vi "simple_qa_agent_sm_template.vi"() -> ()   [LabVIEW 2020]
uses:
  user_interfaces/simple_html_chat_ui/simple_html_chat_ui.lvclass
  models/abstract_llm_base/abstract_llm_base.lvclass
  vectorstore/abstract_vector_base/abstract_vector_base.lvclass
  agent_simple_qa/agent_simple_qa.lvclass
  models/message_text/message_text.lvclass
  <vilib>/addons/_JKI Toolkits/State Machine/_JKI_lib_State_Machine.llb/Select State(s)_err__jki_lib_state_machine.vi
  vectorstore/vector_qdrant/vector_qdrant.lvclass
  D:/petwork/labview-llm-libraries/src/vectorstore/abstract_vector_base/abstract_vector_base.lvclass
  models/llm_openai_chatmodels/llm_openai_chatmodels.lvclass
  D:/petwork/labview-llm-libraries/src/models/abstract_llm_base/abstract_llm_base.lvclass
  models/llm_openai_embedding/llm_openai_embedding.lvclass
  agent_simple_qa_dynamicdata/agent_simple_qa_dynamic.lvclass
  D:/petwork/labview-llm-libraries/src/agent/agent_simple_qa/agent_simple_qa.lvclass
  <vilib>/addons/_JKI Toolkits/State Machine/_JKI_lib_State_Machine.llb/Periodic Trigger__ogtk__JKI-SM__jki_lib_state_machine.vi
  models/message_text/create_text_message.vi
  models/llm_openai_chatmodels/Instantiate_llm_openai.vi
  models/llm_openai_embedding/Instantiate_llm_openai_embed.vi
  agent_simple_qa/poly/ask_your_model.vi
panel:
  in  "new_message":string
  in  "send":bool
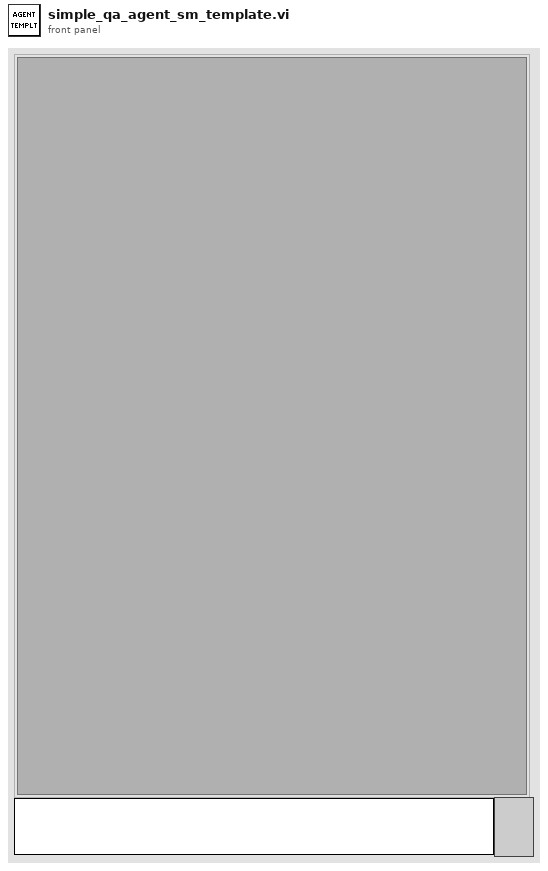
[diagram p1: front panel]
types:
  T1 = enum32{"Invalid", "Standard", "Closed", "Hidden", "Minimized", "Maximized"}
  T2 = enum32{"invalid app kind", "Development System", "Run Time System", "Student Edition", "Embedded LabVIEW", "Evaluation", "Custom"}
  T3 = cluster{"Core":cluster{"Current VI Reference":refnum<vi>, "Close Panel on Exit?":bool}, "Agent":cluster{"UI_Chat":refnum<class "simple_html_chat_ui.lvclass">, "Model_Generative":refnum<class "abstract_llm_base.lvclass">, "Model_Embedding":refnum<class "abstract_llm_base.lvclass">, "Vector Store":refnum<class "abstract_vector_base.lvclass">, "Agent_QA":refnum<class "agent_simple_qa.lvclass">, "last_message":refnum<class "message_text.lvclass">}}
  T4 = cluster{"UI_Chat":refnum<class "simple_html_chat_ui.lvclass">, "Model_Generative":refnum<class "abstract_llm_base.lvclass">, "Model_Embedding":refnum<class "abstract_llm_base.lvclass">, "Vector Store":refnum<class "abstract_vector_base.lvclass">, "Agent_QA":refnum<class "agent_simple_qa.lvclass">, "last_message":refnum<class "message_text.lvclass">}
  T5 = cluster{"Current VI Reference":refnum<vi>, "Close Panel on Exit?":bool}
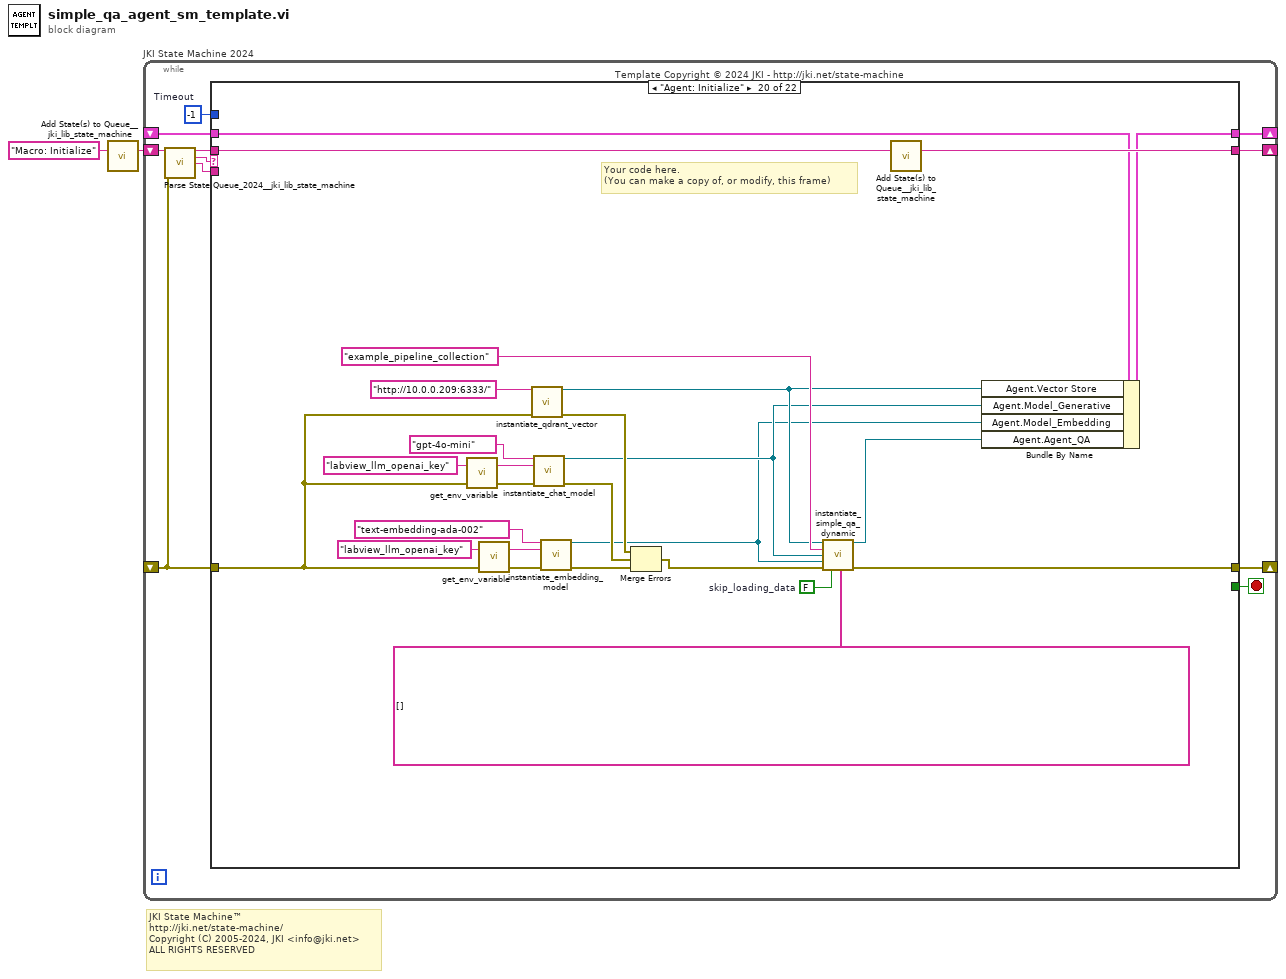
[diagram p0: block diagram]
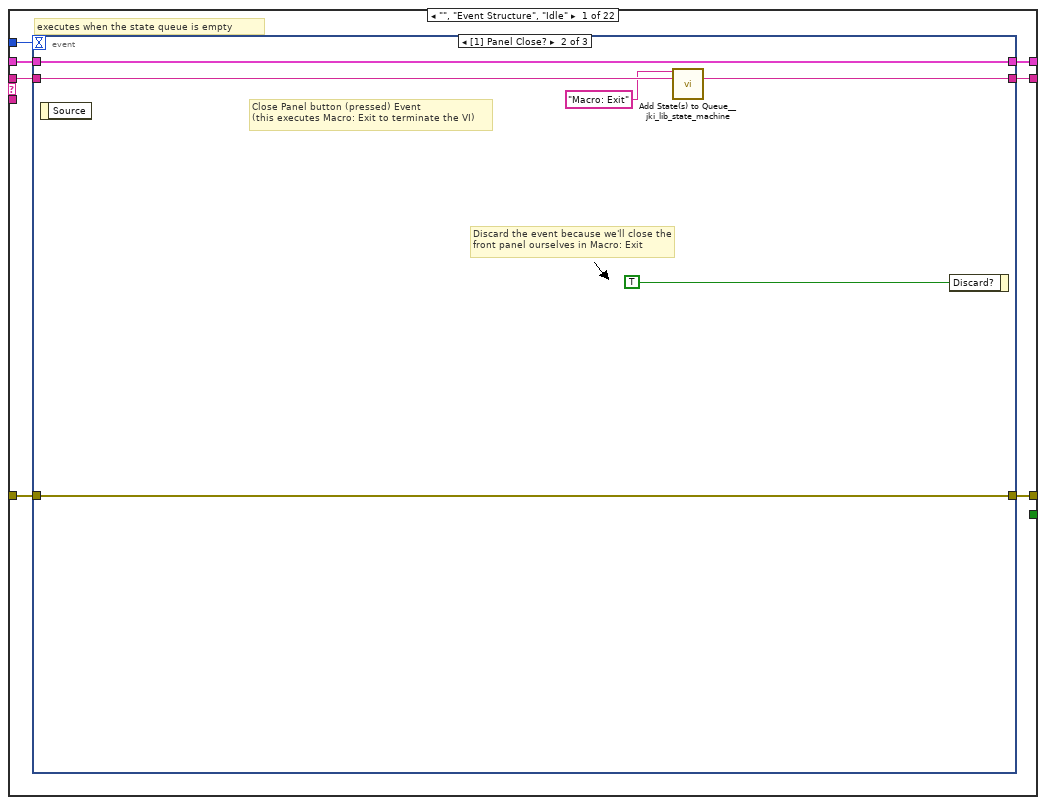
[diagram p2: hidden frame]
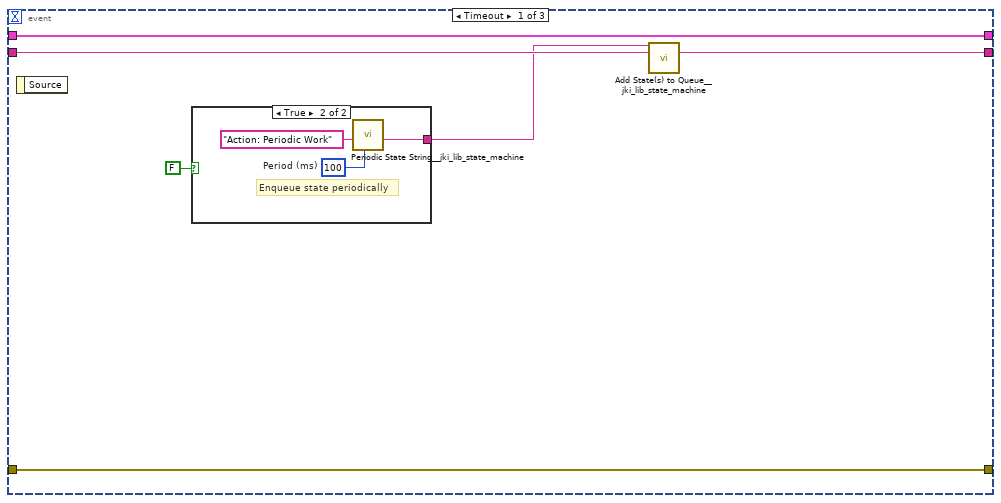
[diagram p3: hidden frame]
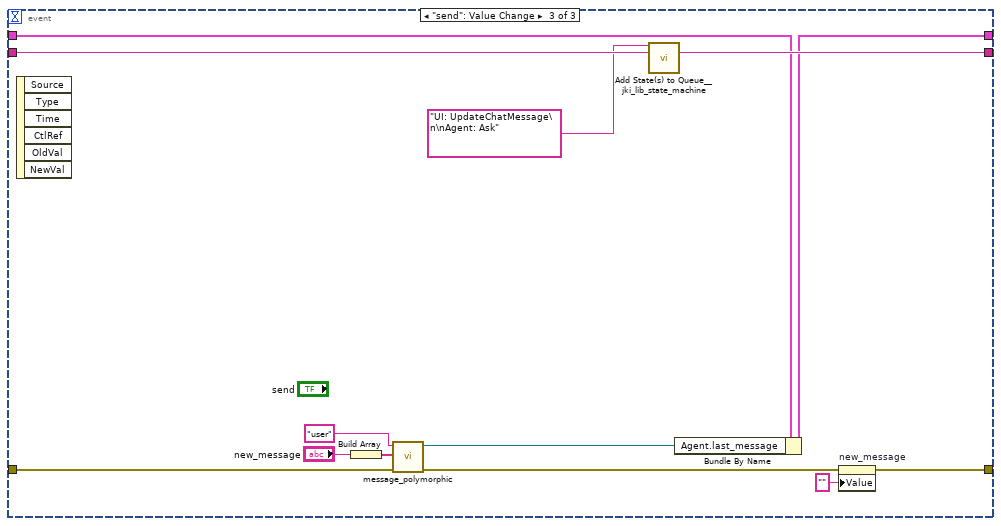
[diagram p5: hidden frame]
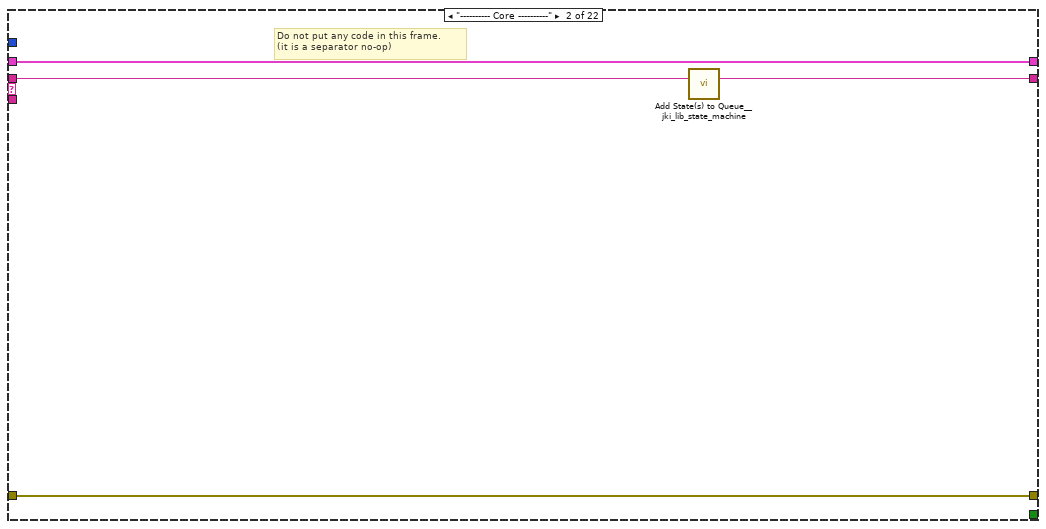
[diagram p6: hidden frame]
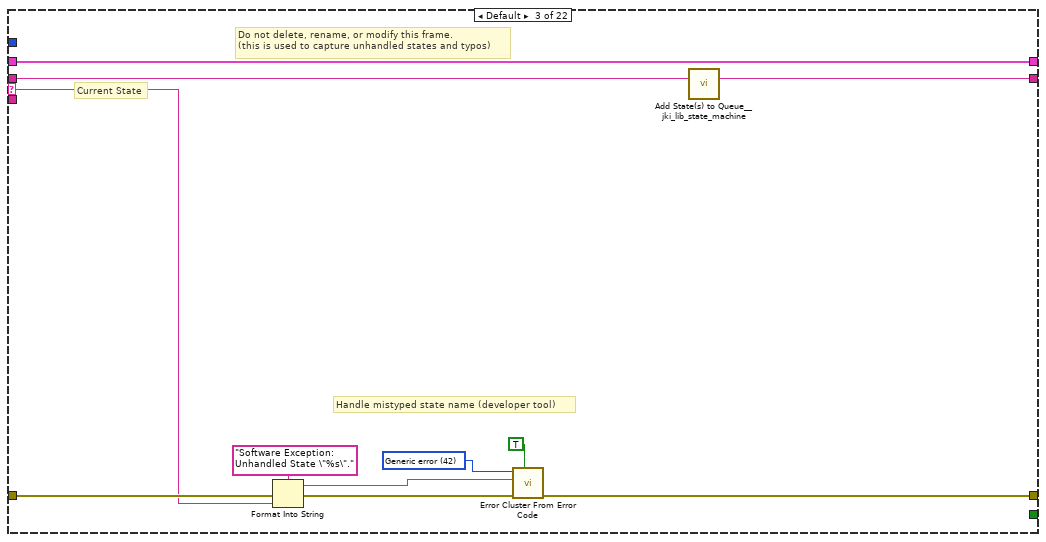
[diagram p7: hidden frame]
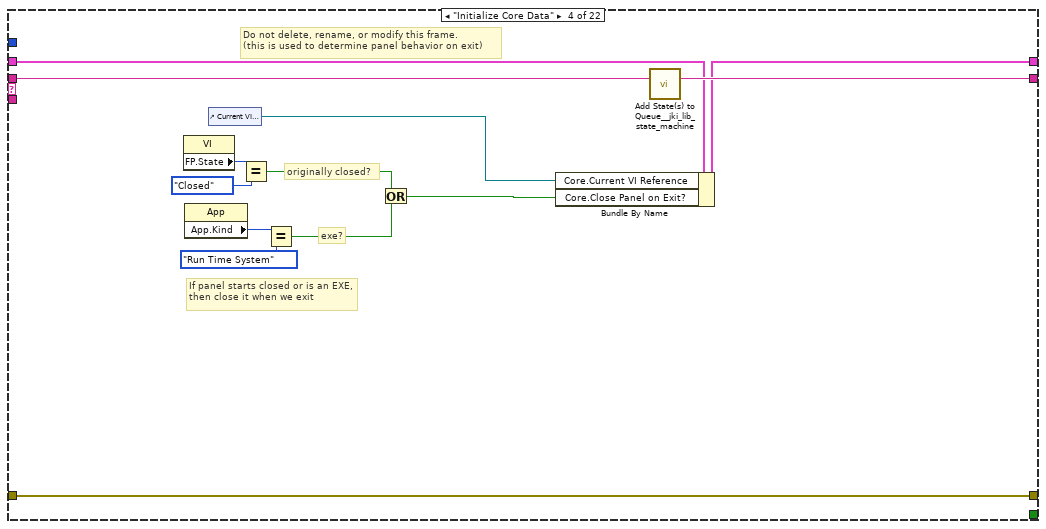
[diagram p8: hidden frame]
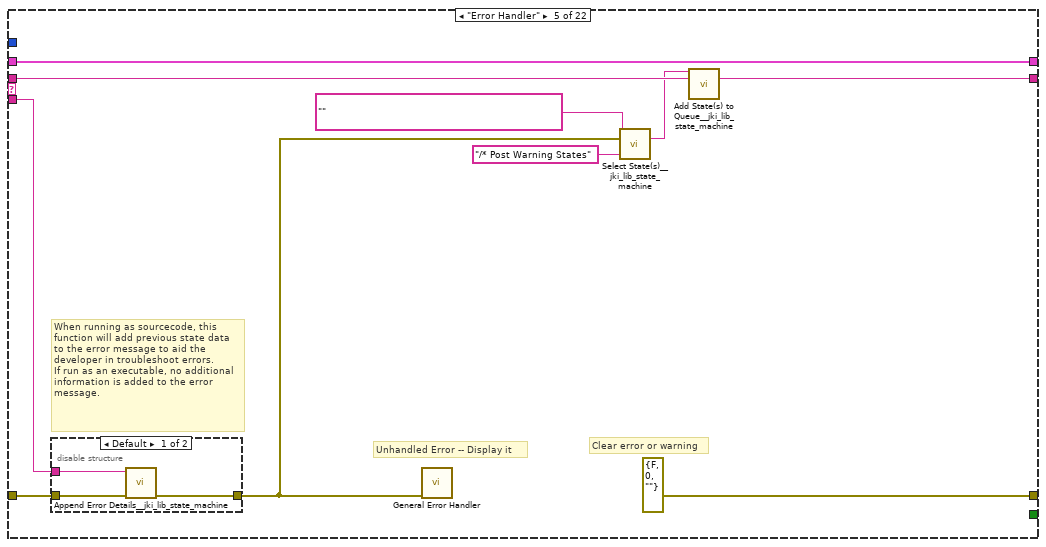
[diagram p9: hidden frame]
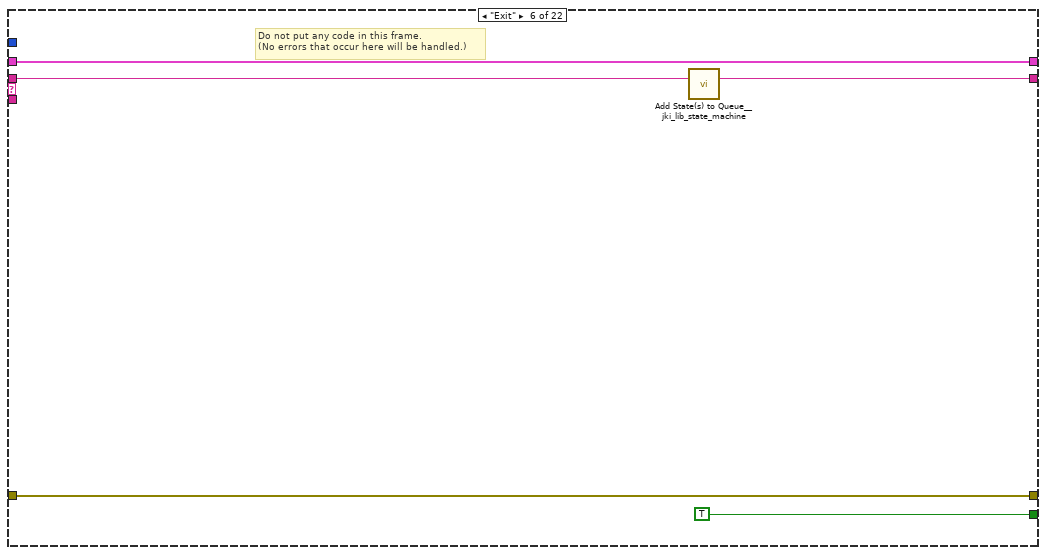
[diagram p11: hidden frame]
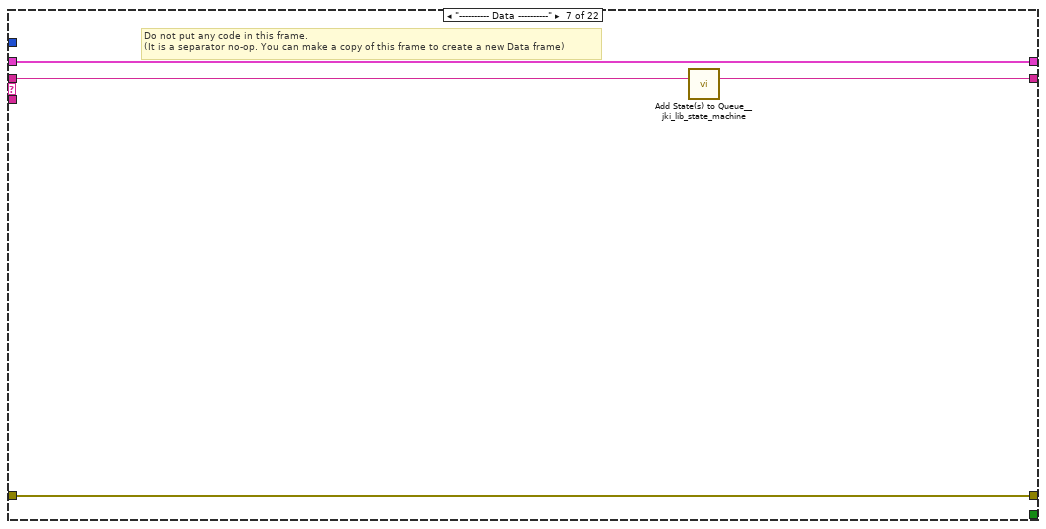
[diagram p12: hidden frame]
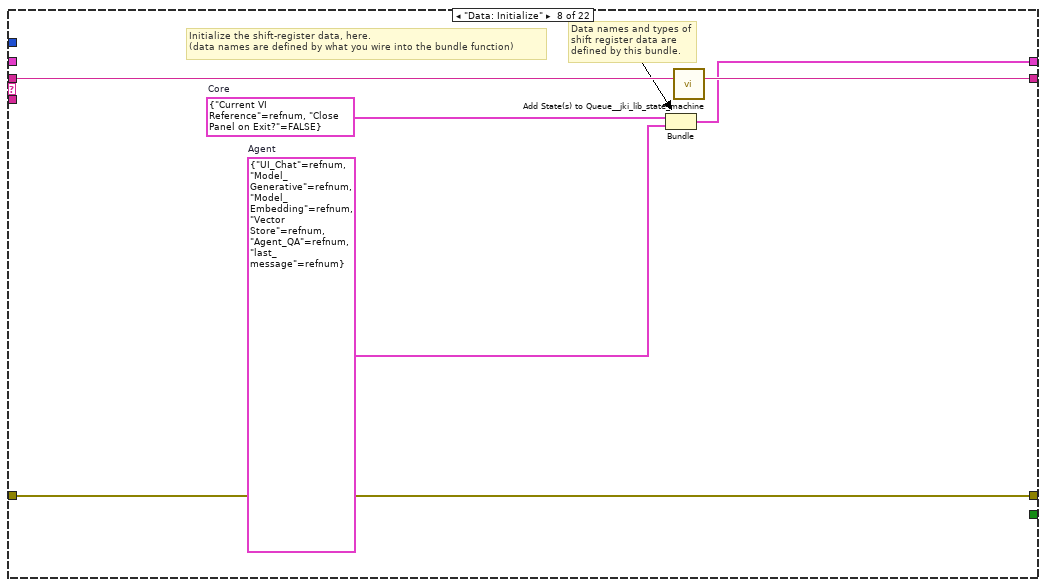
[diagram p13: hidden frame]
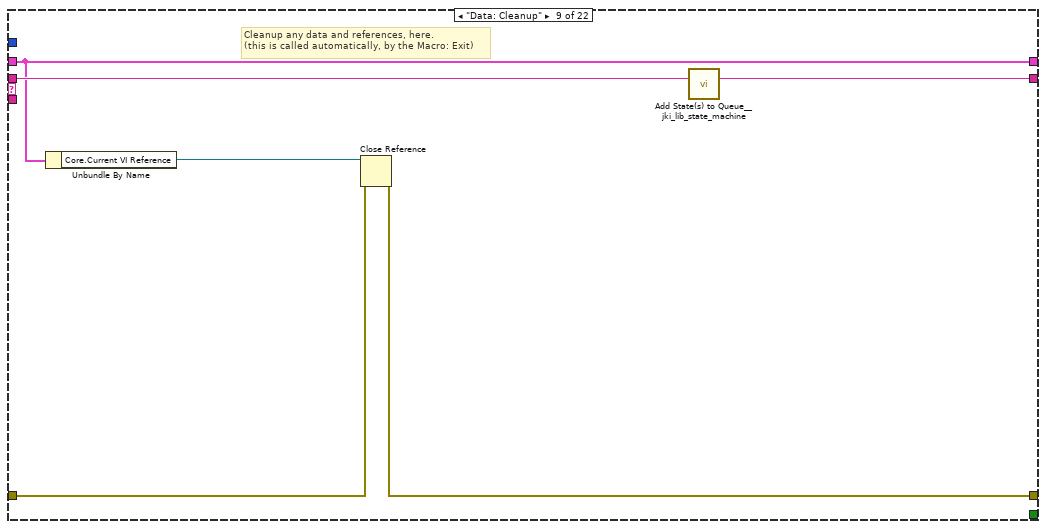
[diagram p14: hidden frame]
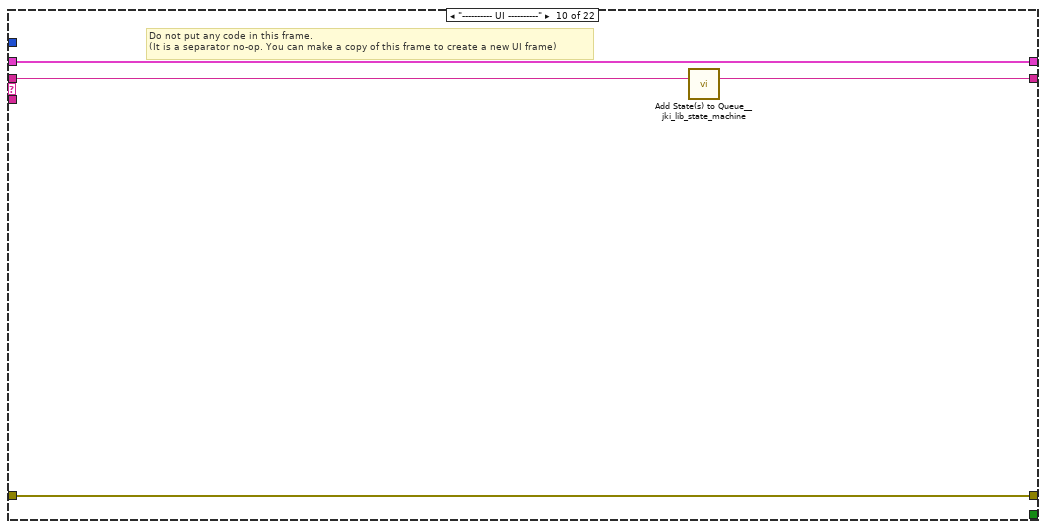
[diagram p15: hidden frame]
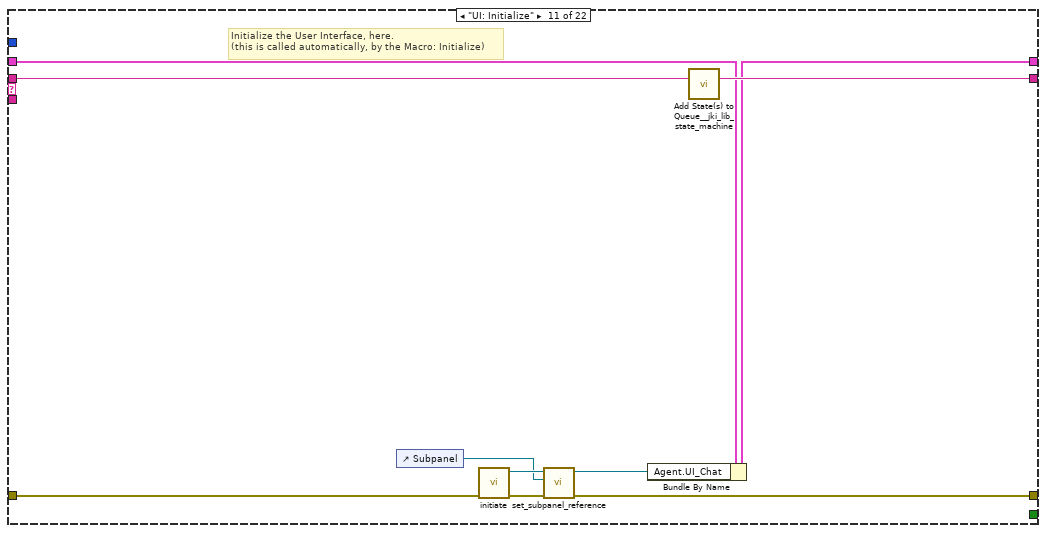
[diagram p16: hidden frame]
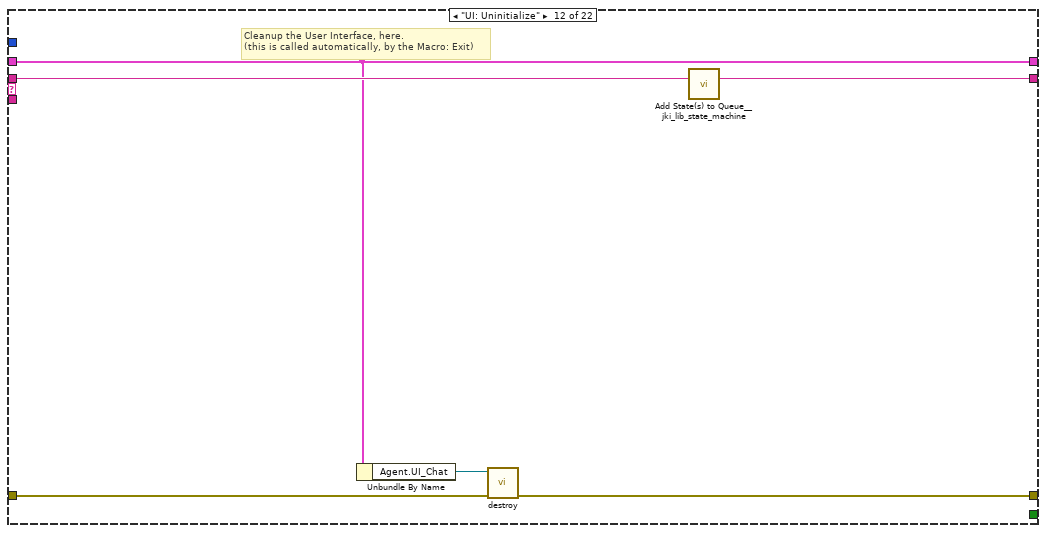
[diagram p17: hidden frame]
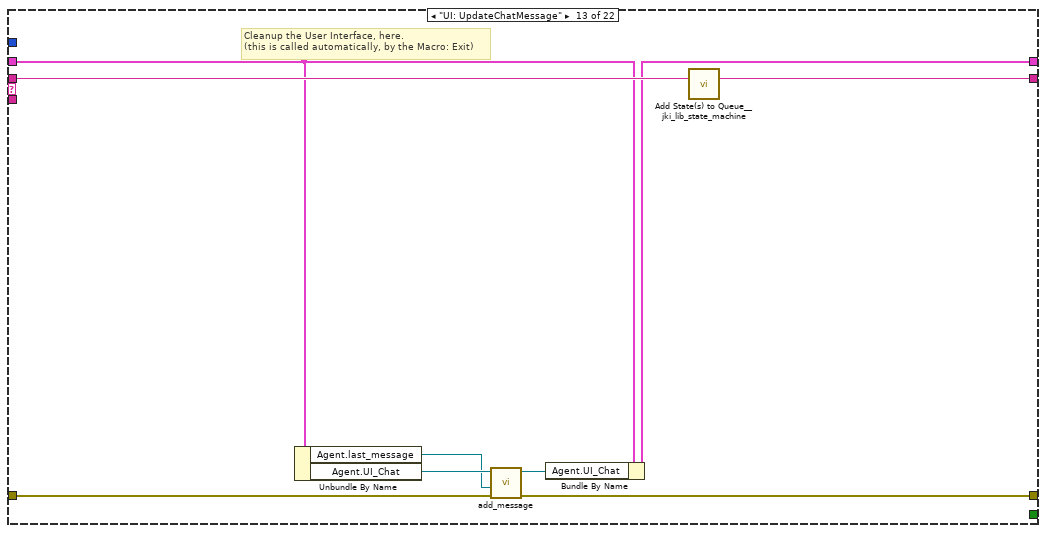
[diagram p18: hidden frame]
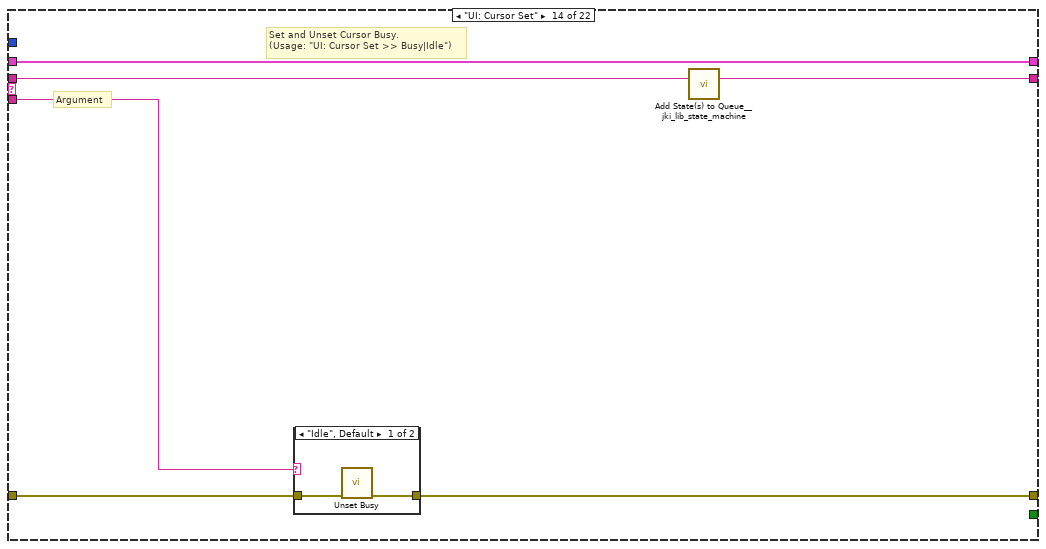
[diagram p19: hidden frame]
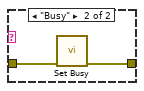
[diagram p20: hidden frame]
diagram:
  # "JKI State Machine™\nhttp://jki.net/state-machine/\nCopyright (C) 2005-2024, JKI <info@jki.net>\nALL RIGHTS RESERVED"
  n1 = call <vilib>:"Add State(s) to Queue__jki_lib_state_machine.vi"("State(s) in (\"\")"="Macro: Initialize") -> ("States Out"=w2:string)  [unwired: 14 in]
  n2 = while "JKI State Machine 2024" {
    shift-right: [w6] -> _
    shift-left: _ -> [w5]
    shift-right: [w9] -> _
    shift-left: _ -> [w3]
    shift-right: [w8] -> _
    shift-left: w2 -> [w10]
    stop <- w7 stop-if-true
    w4 = -1  # Timeout
    # "Template Copyright © 2024 JKI - http://jki.net/state-machine"
    n3 = call <vilib>:"Parse State Queue_2024__jki_lib_state_machine.vi"("State Queue"=w10, "Error In (no error)"=w3) -> ("Remaining States"=w12:string, "Current State"=w13:string, "Arguments"=w11:string)  [unwired: 11 in]
    n4 = case shown="\"Agent: Initialize\"" w13 {
      selector: w13 -> [_ _ w53 _ _ _ _ _ _ _ _ _ _ _ _ _ _ _ _ _ _ _]
      tunnel: w12 -> [w20 w52 w57 w76 w86 w95 w99 w105 w111 w115 w125 w131 w140 w146 w157 w226 w231 w240 w244 w268 w280 w291]
      tunnel: w11 -> [_ _ _ _ w82 _ _ _ _ _ _ _ _ w141 w151 _ _ _ _ _ _ _]
      tunnel: w5 -> [w18 w49 w55 w69 w77 w93 w96 _ w106 w112 w118 w129 w135 w144 w153 w223 w228 w238 w241 w250 w278 w286]
      tunnel: [w17 w50 w59 w73 errorcluster {"status"=FALSE, "code"=0, "source"=""} ("error out") w92 w97 w102 w107 w113 w119 w127 w137 w142 w154 w224 w229 w235 w242 w256 w272 w287] -> w9
      tunnel: w3 -> [w14 w50 w58 w73 w83 w92 w97 w102 w108 w113 w120 w128 w138 w143 w155 w224 w229 w235 w242 w254 w276 w288]
      tunnel: [w19 w51 w56 w75 w85 w94 w98 w104 w110 w114 w124 w130 w139 w145 w156 w225 w230 w239 w243 w267 w279 w290] -> w8
      tunnel: [_ _ _ _ _ TRUE _ _ _ _ _ _ _ _ _ _ _ _ _ _ _ _] -> w7
      tunnel: [w16 w49 w55 w74 w77 w93 w96 w103 w106 w112 w117 w129 w134 w144 w153 w223 w228 w238 w241 w249 w278 w284] -> w6
      tunnel: w4 -> [w15 _ _ _ _ _ _ _ _ _ _ _ _ _ _ _ _ _ _ _ _ _]
      frame "", "Event Structure", "Idle" {
        # "executes when the state queue is empty"
        n5 = event shown="[1] Panel Close?" {
          selector: _ -> [_ _ _]
          dyn-events: _ -> [_ _ _]
          timeout: w15 -> [_ _ _]
          tunnel: w20 -> [w26 w35 w48]
          tunnel: [w25 w34 w47] -> w19
          tunnel: w18 -> [w23 w32 w41]
          tunnel: [w24 w33 w37] -> w17
          tunnel: w14 -> [w24 w33 w43]
          tunnel: [w23 w32 w39] -> w16
          event Timeout {
            n6 = event-data() -> ()  [unwired: 1 in, 1 out]
            n7 = case shown="True" FALSE {
              tunnel: [_ w29] -> w22
              frame False {
              }
              frame True {
                w27 = u32 100  # Period (ms)
                # "Enqueue state periodically"
                n8 = call <vilib>:"Periodic State String__jki_lib_state_machine.vi"("Period (ms)"=w27, "State"="Action: Periodic Work") -> ("State Out"=w29:string)  [unwired: 9 in]
              }
            }
            n9 = call <vilib>:"Add State(s) to Queue__jki_lib_state_machine.vi"("State(s) in Front (\"\")"=w22, "State(s) in (\"\")"=w26) -> ("States Out"=w25:string)  [unwired: 13 in]
          }
          event Panel Close? {
            # "Discard the event because we'll close the front panel ourselves in Macro: Exit"
            # "Close Panel button (pressed) Event\n(this executes Macro: Exit to terminate the VI)"
            n10 = event-data() -> ()  [unwired: 1 in, 1 out]
            n11 = call <vilib>:"Add State(s) to Queue__jki_lib_state_machine.vi"("State(s) in Front (\"\")"="Macro: Exit", "State(s) in (\"\")"=w35) -> ("States Out"=w34:string)  [unwired: 13 in]
            n12 = event-data("Discard?"=TRUE) -> ()  [unwired: 1 in, 1 out]
          }
          event "send": Value Change {
            n13 = event-data() -> ()  [unwired: 1 in, 6 out]
            n14 = Build Array("new_message") -> (w44:string[])
            n15 = call-poly "message_polymorphic.vi"("error in (no error)"=w43, "content"=w44, "role"="user") -> ("error out"=w38:errorcluster, "message_text out"=w40:refnum<class "message_text.lvclass">)  [unwired: 7 in]
            n16 = call <vilib>:"Add State(s) to Queue__jki_lib_state_machine.vi"("State(s) in Front (\"\")"="UI: UpdateChatMessage\n\nAgent: Ask", "State(s) in (\"\")"=w48) -> ("States Out"=w47:string)  [unwired: 13 in]
            n17 = Bundle By Name(cluster=w41, "Agent.last_message"=w40) -> (w39:T3)
            n18 = property on="new_message" class="Str"(error in=w38, "Value"="" ("new_message")) -> (error out=w37:errorcluster)  [unwired: 1 in, 1 out]
          }
        }
      }
      frame "---------- Core ----------" {
        # "Do not put any code in this frame.\n(it is a separator no-op)"
        n19 = call <vilib>:"Add State(s) to Queue__jki_lib_state_machine.vi"("State(s) in (\"\")"=w52) -> ("States Out"=w51:string)  [unwired: 14 in]
      }
      frame Default {
        w62 = 42 items=["No error", "Argument error", "Memory is full", "Out of zone", "End of file", "File already open", "Generic file I/O error", "File not found", "File permission error", "Disk is full", "Duplicate path", "Too many files open", "System feature not enabled", "Resource file not found", "Cannot add resource", "Resource not found", "Image not found", "Image memory error", "Pen does not exist", "Config type invalid", "Config token not found", "Config parse error", "Config memory error", "Bad external code format", "Bad external code offset", "External code not present", "Null window", "Destroy window error", "Null menu", "Print aborted", "Bad print record", "Print driver error", "Windows error during printing", "Memory error during printing", "Print dialog error", "Generic print error", "Invalid device refnum", "Device not found", "Device parameter error", "Device unit error", "Cannot open device", "Device call aborted", "Generic error", "Cancelled by user", "Object ID too low", "Object ID too high", "Object not in heap", "Unknown heap", "Unknown object (invalid DefProc)", "Unknown object (DefProc not in table)", "Message out of range", "Invalid (null) method", "Unknown message", "Manager call not supported", "Bad address", "Network operation in progress", "Network operation timed out", "Connection is busy", "Network attribute not supported", "Network error", "Address in use", "System out of memory", "Connection aborted", "Connection refused", "Not connected", "Already connected", "Connection closed", "Initialization error (interapplication manager)", "Bad occurrence", "Wait on unbound occurrence handler", "Occurrence queue overflow", "Datalog type conflict", "Unused", "Unrecognized type (interapplication manager)", "Memory corrupt", "Failed to make temporary DLL", "Old CIN version", "Drag socket not found", "Failed to load drop-object", "Failed to register OLE object", "Failed to release OLE object", "Format specifier type mismatch", "Unknown format specifier", "Too few format specifiers", "Too many format specifiers", "Scan failed", "Newer CIN version", "Error converting to variant", "Runtime menu error", "Password tampered", "Variant attribute not found", "Incompatible variant data type", "Event data is not available", "Event Store is not present", "Occurrence is not found", "Event Queue is not created", "Event info is not available", "Refnum passed is NULL", "Error retrieving Class GUID", "Error retrieving CoClass GUID", "Error retrieving TypeLib GUID.", "Bad built application magic bytes.", "Specific driver is different from the specific driver associated with the Logical Name.", "There is no session opened to the class driver.", "Max Error", "MAX - Error with config objects", "MAX - Error loading configuration", "MAX - Group not supported"]
        # "Current State"
        # "Do not delete, rename, or modify this frame.\n(this is used to capture unhandled states and typos)"
        # "Handle mistyped state name (developer tool)"
        n20 = Format Into String(format string="Software Exception: Unhandled State \"%s\"." ("message"), error in=w58, w53) -> (resulting string=w61:string, error out=w60:errorcluster)  [unwired: 1 in]
        n21 = call <vilib>:"Error Cluster From Error Code.vi"("show call chain? (False)"=TRUE, "error in (no error)"=w60, "error message (\"\")"=w61, "error code (0)"=w62) -> ("error out"=w59:errorcluster)  [unwired: 5 in]
        n22 = call <vilib>:"Add State(s) to Queue__jki_lib_state_machine.vi"("State(s) in (\"\")"=w57) -> ("States Out"=w56:string)  [unwired: 14 in]
      }
      frame "Initialize Core Data" {
        # "Do not delete, rename, or modify this frame.\n(this is used to determine panel behavior on exit)"
        # "originally closed?"
        # "exe?"
        # "If panel starts closed or is an EXE, then close it when we exit"
        n23 = property class="VI"() -> ("FP.State"=w66:T1)  [unwired: 2 in, 2 out]
        n24 = property class="App"() -> ("App.Kind"=w72:T2)  [unwired: 2 in, 2 out]
        n25 = control-ref of="Current VI Reference"() -> (w67:refnum<vi>)
        n26 = Equal?(x=w66, y=T1."Closed" ("Front Panel Window:State")) -> (x = y?=w64:bool)
        n27 = Equal?(x=w72, y=T2."Run Time System" ("Application:Kind")) -> (x = y?=w70:bool)
        n28 = Or(x=w64, y=w70) -> (x .or. y?=w68:bool)
        n29 = Bundle By Name(cluster=w69, "Core.Current VI Reference"=w67, "Core.Close Panel on Exit?"=w68) -> (w74:T3)
        n30 = call <vilib>:"Add State(s) to Queue__jki_lib_state_machine.vi"("State(s) in (\"\")"=w76) -> ("States Out"=w75:string)  [unwired: 14 in]
      }
      frame "Error Handler" {
        # "Unhandled Error -- Display it"
        # "When running as sourcecode, this function will add previous state data to the error message to aid the developer in troubleshoot errors.\nIf run as an executable, no additional information is added to the error message."
        # "Clear error or warning"
        n31 = disable-structure shown="Default" {
          disable-tunnel: w83 -> [w89 w90]
          disable-tunnel: w82 -> [w88 _]
          disable-tunnel: [w87 w90] -> w81
          frame condition #0 (active) {
            n32 = call <vilib>:"Append Error Details__jki_lib_state_machine.vi"("error in (no error)"=w89, "Previous State and Argument(s)"=w88) -> ("error out"=w87:errorcluster)  [unwired: 9 in]
          }
          frame condition #1 {
          }
        }
        n33 = call <vilib>:"General Error Handler.vi"("error in (no error)"=w81) -> ()  [unwired: 10 in, 5 out]
        n34 = call-poly <vilib>:"Select State(s)__jki_lib_state_machine.vi"("State(s) if True (\"\")"="", "Select"=w81, "State(s) if False (\"\")"="/* Post Warning States") -> ("States Out"=w79:string)  [unwired: 12 in]
        n35 = call <vilib>:"Add State(s) to Queue__jki_lib_state_machine.vi"("State(s) in Front (\"\")"=w79, "State(s) in (\"\")"=w86) -> ("States Out"=w85:string)  [unwired: 13 in]
      }
      frame "Exit" {
        # "Do not put any code in this frame.\n(No errors that occur here will be handled.)"
        n36 = call <vilib>:"Add State(s) to Queue__jki_lib_state_machine.vi"("State(s) in (\"\")"=w95) -> ("States Out"=w94:string)  [unwired: 14 in]
      }
      frame "---------- Data ----------" {
        # "Do not put any code in this frame.\n(It is a separator no-op. You can make a copy of this frame to create a new Data frame)"
        n37 = call <vilib>:"Add State(s) to Queue__jki_lib_state_machine.vi"("State(s) in (\"\")"=w99) -> ("States Out"=w98:string)  [unwired: 14 in]
      }
      frame "Data: Initialize" {
        w100 = T4 {"UI_Chat"=refnum, "Model_Generative"=refnum, "Model_Embedding"=refnum, "Vector Store"=refnum, "Agent_QA"=refnum, "last_message"=refnum}  # Agent
        w101 = T5 {"Current VI Reference"=refnum, "Close Panel on Exit?"=FALSE}  # Core
        # "Data names and types of shift register data are defined by this bundle."
        # "Initialize the shift-register data, here.\n(data names are defined by what you wire into the bundle function)"
        n38 = Bundle("Core"=w101, "Agent"=w100) -> (w103:T3)  [unwired: 1 in]
        n39 = call <vilib>:"Add State(s) to Queue__jki_lib_state_machine.vi"("State(s) in (\"\")"=w105) -> ("States Out"=w104:string)  [unwired: 14 in]
      }
      frame "Data: Cleanup" {
        # "Cleanup any data and references, here.\n(this is called automatically, by the Macro: Exit)"
        n40 = Unbundle By Name(w106) -> ("Core.Current VI Reference"=w109:refnum<vi>)
        n41 = Close Reference(reference=w109, error in (no error)=w108) -> (error out=w107:errorcluster)
        n42 = call <vilib>:"Add State(s) to Queue__jki_lib_state_machine.vi"("State(s) in (\"\")"=w111) -> ("States Out"=w110:string)  [unwired: 14 in]
      }
      frame "---------- UI ----------" {
        # "Do not put any code in this frame.\n(It is a separator no-op. You can make a copy of this frame to create a new UI frame)"
        n43 = call <vilib>:"Add State(s) to Queue__jki_lib_state_machine.vi"("State(s) in (\"\")"=w115) -> ("States Out"=w114:string)  [unwired: 14 in]
      }
      frame "UI: Initialize" {
        # "Initialize the User Interface, here.\n(this is called automatically, by the Macro: Initialize)"
        n44 = control-ref of="Subpanel"() -> (w121:refnum<vi>)
        n45 = call "initiate.vi"("error in (no error)"=w120) -> ("error out"=w123:errorcluster, "simple_html_chat_ui out"=w122:refnum<class "simple_html_chat_ui.lvclass">)  [unwired: 9 in]
        n46 = call "set_subpanel_reference.vi"("error in (no error)"=w123, "Sub Panel"=w121, "simple_html_chat_ui in"=w122) -> ("error out"=w119:errorcluster, "simple_html_chat_ui out"=w116:refnum<class "simple_html_chat_ui.lvclass">)  [unwired: 7 in]
        n47 = Bundle By Name(cluster=w118, "Agent.UI_Chat"=w116) -> (w117:T3)
        n48 = call <vilib>:"Add State(s) to Queue__jki_lib_state_machine.vi"("State(s) in (\"\")"=w125) -> ("States Out"=w124:string)  [unwired: 14 in]
      }
      frame "UI: Uninitialize" {
        # "Cleanup the User Interface, here.\n(this is called automatically, by the Macro: Exit)"
        n49 = Unbundle By Name(w129) -> ("Agent.UI_Chat"=w126:refnum<class "simple_html_chat_ui.lvclass">)
        n50 = call "destroy.vi"("error in (no error)"=w128, "simple_html_chat_ui in"=w126) -> ("error out"=w127:errorcluster)  [unwired: 8 in, 1 out]
        n51 = call <vilib>:"Add State(s) to Queue__jki_lib_state_machine.vi"("State(s) in (\"\")"=w131) -> ("States Out"=w130:string)  [unwired: 14 in]
      }
      frame "UI: UpdateChatMessage" {
        # "Cleanup the User Interface, here.\n(this is called automatically, by the Macro: Exit)"
        n52 = Unbundle By Name(w135) -> ("Agent.last_message"=w132:refnum<class "message_text.lvclass">, "Agent.UI_Chat"=w136:refnum<class "simple_html_chat_ui.lvclass">)
        n53 = call "add_message.vi"("error in (no error)"=w138, "message_text.lvclass"=w132, "simple_html_chat_ui in"=w136) -> ("error out"=w137:errorcluster, "simple_html_chat_ui out"=w133:refnum<class "simple_html_chat_ui.lvclass">)  [unwired: 7 in]
        n54 = Bundle By Name(cluster=w135, "Agent.UI_Chat"=w133) -> (w134:T3)
        n55 = call <vilib>:"Add State(s) to Queue__jki_lib_state_machine.vi"("State(s) in (\"\")"=w140) -> ("States Out"=w139:string)  [unwired: 14 in]
      }
      frame "UI: Cursor Set" {
        # "Argument"
        # "Set and Unset Cursor Busy.\n(Usage: \"UI: Cursor Set >> Busy|Idle\")"
        n56 = case shown="\"Idle\", Default" w141 {
          tunnel: w143 -> [w148 w150]
          tunnel: [w147 w149] -> w142
          frame "Idle", Default {
            n57 = call <vilib>:"Unset Busy.vi"("error in (no error)"=w148) -> ("error out"=w147:errorcluster)  [unwired: 10 in]
          }
          frame "Busy" {
            n58 = call <vilib>:"Set Busy.vi"("error in (no error)"=w150) -> ("error out"=w149:errorcluster)  [unwired: 9 in, 1 out]
          }
        }
        n59 = call <vilib>:"Add State(s) to Queue__jki_lib_state_machine.vi"("State(s) in (\"\")"=w146) -> ("States Out"=w145:string)  [unwired: 14 in]
      }
      frame "UI: Front Panel State" {
        # "Argument"
        # "Set Front Panel Open or Closed\n(Usage: \"UI: Front Panel State >> Open|Close\")"
        n60 = Unbundle By Name(w153) -> ("Core.Current VI Reference"=w152:refnum<vi>)
        n61 = case shown="\"Minimize\", \"Minimized\"" w151 {
          tunnel: w155 -> [w163 w178 w189 w202 w215]
          tunnel: [w165 w179 w191 w204 w217] -> w154
          tunnel: w152 -> [w164 w176 w190 w203 w216]
          frame "Open", "Standard", Default {
            w158 = T1."Standard" ("State")
            n62 = property class="VI"(reference=w164, error in=w163) -> (reference out=w161:refnum<vi>, error out=w162:errorcluster, "FP.State"=w160:T1)
            n63 = Not Equal?(x=w160, y=w158) -> (x != y?=w159:bool)
            n64 = case shown="True" w159 {
              tunnel: [w169 w171] -> w165
              tunnel: w162 -> [w168 w171]
              tunnel: w161 -> [w167 _]
              tunnel: w158 -> [w166 _]
              frame True {
                n65 = invoke class="VI" method="FP.Open"(reference=w167, error in=w168, "Activate"=TRUE, "State"=w166) -> (error out=w169:errorcluster)  [unwired: 1 in, 4 out]
              }
              frame False {
              }
            }
          }
          frame "Close", "Closed" {
            n66 = property class="VI"(reference=w176, error in=w178) -> (reference out=w175:refnum<vi>, error out=w177:errorcluster, "FP.State"=w173:T1)
            n67 = Not Equal?(x=w173, y=T1."Closed" ("Front Panel Window:State")) -> (x != y?=w172:bool)
            n68 = case shown="True" w172 {
              tunnel: [w180 w183] -> w179
              tunnel: w177 -> [w180 w182]
              tunnel: w175 -> [_ w181]
              frame False {
              }
              frame True {
                n69 = invoke class="VI" method="FP.Close"(reference=w181, error in=w182) -> (error out=w183:errorcluster)  [unwired: 1 in, 2 out]
              }
            }
          }
          frame "Hidden", "Hide" {
            w184 = T1."Hidden" ("State")
            n70 = property class="VI"(reference=w190, error in=w189) -> (reference out=w187:refnum<vi>, error out=w188:errorcluster, "FP.State"=w186:T1)
            n71 = Not Equal?(x=w186, y=w184) -> (x != y?=w185:bool)
            n72 = case shown="True" w185 {
              tunnel: [w195 w196] -> w191
              tunnel: w188 -> [w194 w196]
              tunnel: w187 -> [w193 _]
              tunnel: w184 -> [w192 _]
              frame True {
                n73 = invoke class="VI" method="FP.Open"(reference=w193, error in=w194, "State"=w192) -> (error out=w195:errorcluster)  [unwired: 2 in, 4 out]
              }
              frame False {
              }
            }
          }
          frame "Minimize", "Minimized" {
            w197 = T1."Minimized" ("State")
            n74 = property class="VI"(reference=w203, error in=w202) -> (reference out=w200:refnum<vi>, error out=w201:errorcluster, "FP.State"=w199:T1)
            n75 = Not Equal?(x=w199, y=w197) -> (x != y?=w198:bool)
            n76 = case shown="True" w198 {
              tunnel: [w208 w209] -> w204
              tunnel: w201 -> [w207 w209]
              tunnel: w200 -> [w206 _]
              tunnel: w197 -> [w205 _]
              frame True {
                n77 = invoke class="VI" method="FP.Open"(reference=w206, error in=w207, "State"=w205) -> (error out=w208:errorcluster)  [unwired: 2 in, 4 out]
              }
              frame False {
              }
            }
          }
          frame "Maximize", "Maximized" {
            w210 = T1."Maximized" ("State")
            n78 = property class="VI"(reference=w216, error in=w215) -> (reference out=w213:refnum<vi>, error out=w214:errorcluster, "FP.State"=w212:T1)
            n79 = Not Equal?(x=w212, y=w210) -> (x != y?=w211:bool)
            n80 = case shown="True" w211 {
              tunnel: [w221 w222] -> w217
              tunnel: w214 -> [w220 w222]
              tunnel: w213 -> [w219 _]
              tunnel: w210 -> [w218 _]
              frame True {
                n81 = invoke class="VI" method="FP.Open"(reference=w219, error in=w220, "State"=w218) -> (error out=w221:errorcluster)  [unwired: 2 in, 4 out]
              }
              frame False {
              }
            }
          }
        }
        n82 = call <vilib>:"Add State(s) to Queue__jki_lib_state_machine.vi"("State(s) in (\"\")"=w157) -> ("States Out"=w156:string)  [unwired: 14 in]
      }
      frame "---------- Macro ----------" {
        # "Do not put any code in this frame.\n(It is a separator no-op. You can make a copy of this frame to create a new Macro frame)"
        n83 = call <vilib>:"Add State(s) to Queue__jki_lib_state_machine.vi"("State(s) in (\"\")"=w226) -> ("States Out"=w225:string)  [unwired: 14 in]
      }
      frame "Macro: Initialize" {
        w227 = "Data: Initialize\nInitialize Core Data\nUI: Initialize\nUI: Front Panel State >> Open\n\nAgent: Initialize"  # Data: Initialize Initialize Core Data UI: Initialize UI: Front Panel State >> Open  Agent: Initialize
        # "Initialization Macro\n(This is called once, when the VI starts)"
        n84 = call <vilib>:"Add State(s) to Queue__jki_lib_state_machine.vi"("State(s) in Front (\"\")"=w227, "State(s) in (\"\")"=w231) -> ("States Out"=w230:string)  [unwired: 13 in]
      }
      frame "Macro: Exit" {
        # "Exit Macro\n(This is called once, when the VI exits)"
        n85 = Unbundle By Name(w238) -> ("Core.Close Panel on Exit?"=w233:bool)
        n86 = call <vilib>:"Conditional State String__jki_lib_state_machine.vi"("Do State(s)?"=w233, "State"="UI: Front Panel State >> Close") -> ("State Out"=w232:string)  [unwired: 7 in]
        n87 = call <vilib>:"Add State(s) to Queue__jki_lib_state_machine.vi"("State(s) in (\"\")"=w232, "State(s) at Back (\"\")"="UI: Uninitialize\nData: Cleanup\n\nAgent: Close\n\nExit") -> ("States Out"=w236:string)  [unwired: 13 in]
        n88 = call <vilib>:"Add State(s) to Queue__jki_lib_state_machine.vi"("State(s) in Front (\"\")"=w236, "State(s) in (\"\")"=w240) -> ("States Out"=w239:string)  [unwired: 13 in]
      }
      frame "----------Agents----------" {
        # "Template Separator\n(You can make a copy of, or modify, this frame)"
        n89 = call <vilib>:"Add State(s) to Queue__jki_lib_state_machine.vi"("State(s) in (\"\")"=w244) -> ("States Out"=w243:string)  [unwired: 14 in]
      }
      frame "Agent: Initialize" {
        w257 = FALSE  # skip_loading_data
        # "Your code here.\n(You can make a copy of, or modify, this frame)"
        n90 = call "get_env_variable.vi"("Environment Variable Name"="labview_llm_openai_key") -> ("Value"=w264:string)  [unwired: 1 in, 1 out]
        n91 = call "get_env_variable.vi"("Environment Variable Name"="labview_llm_openai_key") -> ("Value"=w259:string)  [unwired: 1 in, 1 out]
        n92 = call "instantiate_qdrant_vector.vi"("host_url"="http://10.0.0.209:6333/", "error in"=w254) -> ("vector_qdrant out"=w247:refnum<class "vector_qdrant.lvclass">, "error out"=w252:errorcluster)  [unwired: 12 in]
        n93 = call-poly "instantiate_chat_model.vi"("model_name"="gpt-4o-mini", "openai_key"=w264, "error in (no error)"=w254) -> ("llm_openai out"=w246:refnum<class "llm_openai_chatmodels.lvclass">, "error out"=w251:errorcluster)  [unwired: 11 in]
        n94 = call-poly "instantiate_embedding_model.vi"("model_name"="text-embedding-ada-002", "openai_key"=w259, "error in (no error)"=w254) -> ("llm_openai_embedding out"=w245:refnum<class "llm_openai_embedding.lvclass">, "error out"=w255:errorcluster)  [unwired: 11 in]
        n95 = Merge Errors(w252, w251, w255) -> (w253:errorcluster)
        n96 = call "instantiate_simple_qa_dynamic.vi"("vectorestore"=w247, "skip_loading_data"=w257, "collection_name"="example_pipeline_collection" ("host_url"), "chat_model"=w246, "embedding_model"=w245, "error in (no error)"=w253, "sources"=string[] [] ("webpages")) -> ("agent_webpage_qa out"=w248:refnum<class "agent_simple_qa_dynamic.lvclass">, "error out"=w256:errorcluster)  [unwired: 7 in]
        n97 = call <vilib>:"Add State(s) to Queue__jki_lib_state_machine.vi"("State(s) in (\"\")"=w268) -> ("States Out"=w267:string)  [unwired: 14 in]
        n98 = Bundle By Name(cluster=w250, "Agent.Vector Store"=w247, "Agent.Model_Generative"=w246, "Agent.Model_Embedding"=w245, "Agent.Agent_QA"=w248) -> (w249:T3)
      }
      frame "Agent: Close" {
        # "Your code here.\n(You can make a copy of, or modify, this frame)"
        n99 = Unbundle By Name(w278) -> ("Agent.Model_Generative"=w269:refnum<class "abstract_llm_base.lvclass">, "Agent.Model_Embedding"=w270:refnum<class "abstract_llm_base.lvclass">, "Agent.Vector Store"=w271:refnum<class "abstract_vector_base.lvclass">, "Agent.Agent_QA"=w277:refnum<class "agent_simple_qa.lvclass">)
        n100 = call-dynamic "destroy.vi"("agent_simple_qa in"=w277, "error in (no error)"=w276) -> ("error out"=w275:errorcluster)  [unwired: 12 in, 1 out]
        n101 = call-dynamic "destroy.vi"("abstract_vector_base in"=w271, "error in (no error)"=w275) -> ("error out"=w274:errorcluster)  [unwired: 12 in, 1 out]
        n102 = call-dynamic "destroy.vi"("error in (no error)"=w274, "abstract_llm_base in"=w270) -> ("error out"=w273:errorcluster)  [unwired: 8 in, 1 out]
        n103 = call-dynamic "destroy.vi"("error in (no error)"=w273, "abstract_llm_base in"=w269) -> ("error out"=w272:errorcluster)  [unwired: 8 in, 1 out]
        n104 = call <vilib>:"Add State(s) to Queue__jki_lib_state_machine.vi"("State(s) in (\"\")"=w280) -> ("States Out"=w279:string)  [unwired: 14 in]
      }
      frame "Agent: Ask" {
        n105 = Unbundle By Name(w286) -> ("Agent.last_message"=w283:refnum<class "message_text.lvclass">, "Agent.Agent_QA"=w289:refnum<class "agent_simple_qa.lvclass">)
        n106 = call-poly "ask_poly.vi"("error in (no error)"=w288, "message_text"=w283, "agent_simple_qa in"=w289) -> ("error out"=w287:errorcluster, "message_text_response"=w282:refnum<class "message_text.lvclass">, "agent_simple_qa out"=w285:refnum<class "agent_simple_qa.lvclass">)  [unwired: 6 in]
        n107 = Bundle By Name(cluster=w286, "Agent.last_message"=w282, "Agent.Agent_QA"=w285) -> (w284:T3)
        n108 = call <vilib>:"Add State(s) to Queue__jki_lib_state_machine.vi"("State(s) in Front (\"\")"="UI: UpdateChatMessage" ("State(s) in Front (\"\")"), "State(s) in (\"\")"=w291) -> ("States Out"=w290:string)  [unwired: 13 in]
      }
    }
  }
